vi "Curtin1_ReadWriteView.vi"(8 "X_High":dbl, 9 "X_Low":dbl, 11 "Task":enum16{"Read", "Save"}(ring)) -> (0 "X_High out":dbl, 1 "X_Low out":dbl, 3 "View":T1={"Alerts"=FALSE, "Log X Axis"=TRUE, "dB scale"=TRUE, "Averaging"=TRUE, "Fade"=0.8181818181818182, "Centroids?"=TRUE})   [LabVIEW 2022 SP3]
uses:
  Mic/Mic_Global.vi
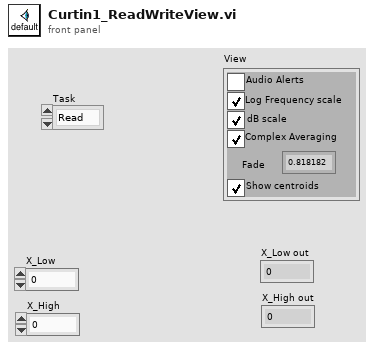
[diagram p1: front panel]
types:
  T1 = cluster{"Alerts":bool, "Log X Axis":bool, "dB scale":bool, "Averaging":bool, "Fade":dbl, "Centroids?":bool}
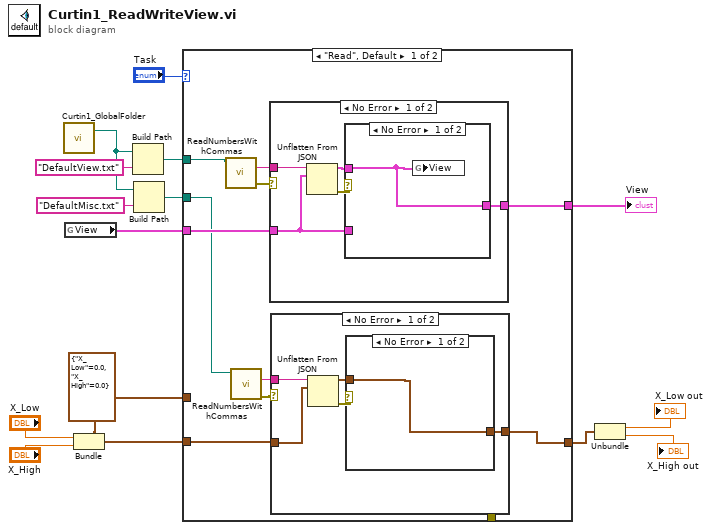
[diagram p0: block diagram]
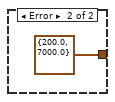
[diagram p2: hidden frame]
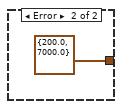
[diagram p3: hidden frame]
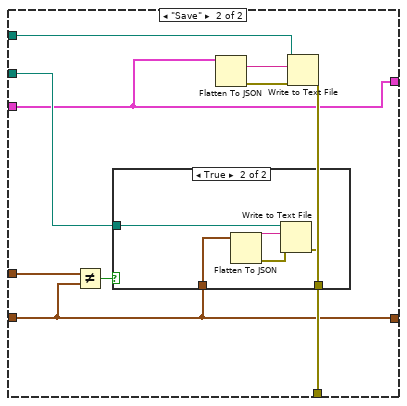
[diagram p6: hidden frame]
diagram:
  w2 = cluster{"X_Low":dbl, "X_High":dbl} {"X_Low"=0.0, "X_High"=0.0} ("output cluster")
  n1 = call "Curtin1_GlobalFolder.vi"() -> ("LabVIEW Data Path"=w8:path)  [unwired: 1 in, 1 out]
  n2 = global read "Mic_Global.vi" "View"() -> (w7:T1)
  n3 = Bundle(cluster=w2, "X_Low"="X_Low", "X_High"="X_High") -> (w10:cluster{"X_Low":dbl, "X_High":dbl})
  n4 = Build Path(base path=w8, name or relative path="DefaultView.txt") -> (appended path=w14:path)
  n5 = Build Path(base path=w8, name or relative path="DefaultMisc.txt") -> (appended path=w6:path)
  n6 = case shown="\"Read\", Default" "Task" {
    tunnel: w14 -> [w18 w48]
    tunnel: [_ w47] -> _
    tunnel: w10 -> [w24 w43]
    tunnel: w7 -> [w25 w42]
    tunnel: w6 -> [w19 w46]
    tunnel: [w23 w43] -> w5
    tunnel: w2 -> [_ w44]
    tunnel: [w22 w42] -> w1
    frame "Read", Default {
      n7 = call "ReadNumbersWithCommas.vi"("file (use dialog)"=w18) -> ("error out"=w16:errorcluster, "text"=w17:string)  [unwired: 7 in, 2 out]
      n8 = call "ReadNumbersWithCommas.vi"("file (use dialog)"=w19) -> ("error out"=w21:errorcluster, "text"=w20:string)  [unwired: 7 in, 2 out]
      n9 = case shown="No Error" w16 {
        tunnel: w17 -> [w38 _]
        tunnel: w25 -> [w34 w41]
        tunnel: [w35 w41] -> w22
        frame No Error {
          n10 = Unflatten From JSON(JSON string=w38, type and defaults=w34) -> (value=w36:T1, error out=w37:errorcluster)  [unwired: 5 in]
          n11 = case shown="No Error" w37 {
            tunnel: w36 -> [w39 _]
            tunnel: [w39 w40] -> w35
            tunnel: w34 -> [_ w40]
            frame No Error {
              n12 = global write "Mic_Global.vi" "View"(w39) -> ()
            }
            frame Error {
            }
          }
        }
        frame Error {
        }
      }
      n13 = case shown="No Error" w21 {
        tunnel: w20 -> [w30 _]
        tunnel: w24 -> [w27 _]
        tunnel: [w26 cluster{"X_Low":dbl, "X_High":dbl} {"X_Low"=200.0, "X_High"=7000.0} ("output cluster")] -> w23
        frame No Error {
          n14 = Unflatten From JSON(JSON string=w30, type and defaults=w27) -> (value=w28:cluster{"X_Low":dbl, "X_High":dbl}, error out=w29:errorcluster)  [unwired: 5 in]
          n15 = case shown="No Error" w29 {
            tunnel: w28 -> [w31 _]
            tunnel: [w31 cluster{"X_Low":dbl, "X_High":dbl} {"X_Low"=200.0, "X_High"=7000.0} ("output cluster")] -> w26
            frame No Error {
            }
            frame Error {
            }
          }
        }
        frame Error {
        }
      }
    }
    frame "Save" {
      n16 = Not Equal?(x=w44, y=w43) -> (x != y?=w45:bool)
      n17 = case shown="True" w45 {
        tunnel: w46 -> [_ w53]
        tunnel: w43 -> [_ w52]
        tunnel: [_ w51] -> _
        frame False {
        }
        frame True {
          n18 = Flatten To JSON(anything=w52) -> (JSON string=w54:string, 11:w55:errorcluster)  [unwired: 2 in]
          n19 = Write to Text File(file (use dialog)=w53, text=w54, error in=w55) -> (error out=w51:errorcluster)  [unwired: 1 in, 2 out]
        }
      }
      n20 = Flatten To JSON(anything=w42) -> (JSON string=w50:string, 11:w49:errorcluster)  [unwired: 2 in]
      n21 = Write to Text File(file (use dialog)=w48, text=w50, error in=w49) -> (error out=w47:errorcluster)  [unwired: 1 in, 2 out]
    }
  }
  "View" <- w1
  n22 = Unbundle(w5) -> ("X_Low"=→"X_Low out":dbl, "X_High"=→"X_High out":dbl)
